vi "Next Step.vi"(8 "error in (no error)":errorcluster, 11 "Continuous.lvclass in":refnum<class "Continuous.lvclass">) -> (0 "error out":errorcluster, 1 "Step #":u32, 2 "actual position":dbl, 3 "Continuous.lvclass out":refnum<class "Continuous.lvclass">)   [LabVIEW 2012, in "Continuous.lvclass"]
uses:
  Continuous.lvclass
  Instruments/Magnet/Power Supply/Power Supply.lvclass
  Scanner/Scanner.lvclass
panel:
  in  "Manual Override":bool
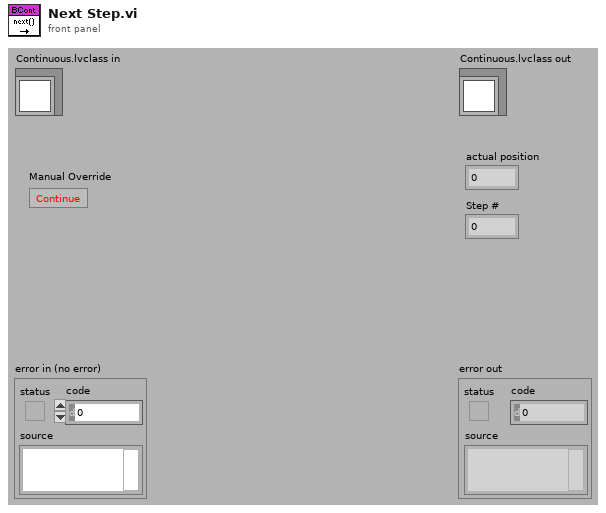
[diagram p1: front panel]
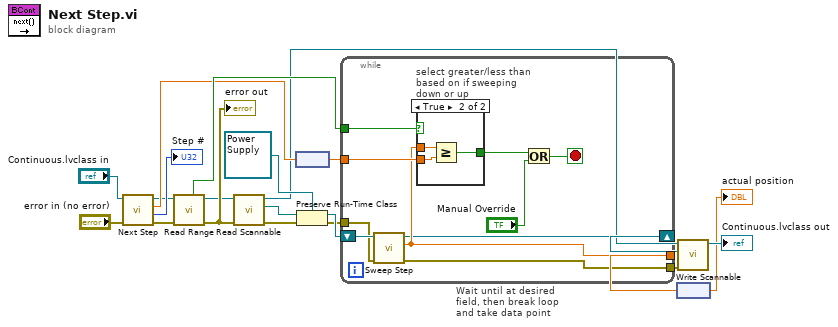
[diagram p0: block diagram]
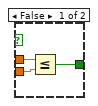
[diagram p2: hidden frame]
diagram:
  n1 = call-parent "Next Step.vi"("error in (no error)"="error in (no error)", "Scanner in"="Continuous.lvclass in") -> ("error out"=w16:errorcluster, "Current Step"=→"Step #":u32, "Current Position"=w17:dbl, "Scanner out"=w14:refnum<class "Continuous.lvclass">)  [unwired: 6 out]
  n2 = call-dynamic "Read Range.vi"("error in (no error)"=w16, "Scanner.lvclass in"=w14) -> ("error out"=w5:errorcluster, "Scanner.lvclass out"=w4:refnum<class "Continuous.lvclass">, "Scanning Up?"=w19:bool)  [unwired: 7 out]
  "error out" <- w5
  n3 = call-dynamic "Read Scannable.vi"("error in (no error)"=w5, "Scanner.lvclass in"=w4) -> ("error out"=w12:errorcluster, "Scannable.lvclass"=w11:refnum<class "Scannable.lvclass">, "Scanner.lvclass out"=w3:refnum<class "Continuous.lvclass">)  [unwired: 7 in]
  n4 = node(w17) -> (w13:dbl[unit])
  n5 = Preserve Run-Time Class(object in=w11, error in=w12, 2:refnum<class "Power Supply.lvclass"> refnum ("Power Supply in")) -> (object out=w9:refnum<class "Power Supply.lvclass">, error out=w6:errorcluster)
  n6 = while "Wait until at desired field, then break loop and take data point" {
    tunnel: [w30] -> w20
    tunnel: w13 -> [w31]
    tunnel: w19 -> [w29]
    shift-right: [w24] -> w8
    shift-left: w9 -> [w25]
    tunnel: [w23] -> w7
    tunnel: w6 -> [w22]
    stop <- w28 stop-if-true
    n7 = call-dynamic "Sweep Step.vi"("error in (no error)"=w22, "Power Supply in"=w25) -> ("error out"=w23:errorcluster, "field"=w30:dbl[unit], "Power Supply out"=w24:refnum<class "Power Supply.lvclass">)  [unwired: 5 in, 2 out]
    n8 = case "select greater/less than based on if sweeping down or up" shown="True" w29 {
      tunnel: w30 -> [w33 w37]
      tunnel: w31 -> [w34 w36]
      tunnel: [w32 w35] -> w27
      frame False {
        n9 = Less Or Equal?(x=w33, y=w34) -> (x <= y?=w32:bool)
      }
      frame True {
        n10 = Greater Or Equal?(x=w37, y=w36) -> (x >= y?=w35:bool)
      }
    }
    n11 = Or(x=w27, y="Manual Override") -> (x .or. y?=w28:bool)
  }
  n12 = node(w20) -> (→"actual position":dbl)
  n13 = call-dynamic "Write Scannable.vi"("error in (no error)"=w7, "Scannable.lvclass"=w8, "Scanner.lvclass in"=w3) -> ("Scanner.lvclass out"=→"Continuous.lvclass out":refnum<class "Continuous.lvclass">)  [unwired: 7 in, 1 out]
